vi "Set Write Mode.vi"(8 "error in (no error)":errorcluster, 10 "Write Mode":T1, 11 "Item Ref in":T2 format="%.0x") -> (0 "error out":errorcluster, 3 "Item Ref out":T2 format="%.0x")   [LabVIEW 2020, in "Modbus Master System Explorer.lvlib"]
uses:
  Modbus Master System Explorer.lvlib
  <vilib>/NI VeriStand/Custom Device API/Custom Device Item Ref.ctl
  Shared/Write Mode.ctl
  Shared/Constants.vi
  <vilib>/NI VeriStand/Custom Device API/Set Item Property (U16).vi
  Shared/Modbus Master Shared.lvlib
  <vilib>/NI VeriStand/Custom Device API/Custom Device API.lvlib
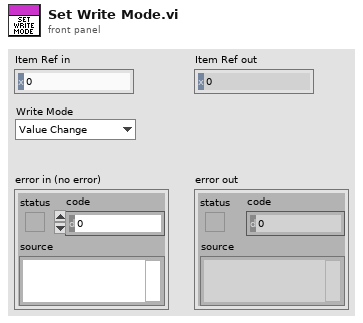
[diagram p1: front panel]
types:
  T1 = typedef "Modbus Master Shared.lvlib/Write Mode.ctl" = enum16{"Value Change", "Interval"}
  T2 = typedef "Custom Device API.lvlib/Custom Device Item Ref.ctl" = u64
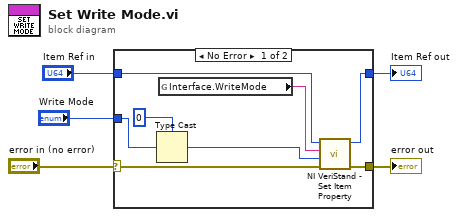
[diagram p0: block diagram]
diagram:
  n1 = case shown="No Error" "error in (no error)" {
    selector: "error in (no error)" -> [w12 w14]
    tunnel: "Item Ref in" -> [w11 w15]
    tunnel: [w10 w14] -> w3
    tunnel: [w9 w15] -> w2
    tunnel: "Write Mode" -> [w7 _]
    frame No Error {
      n2 = Type Cast(type=u16 0 ("Value"), x=w7) -> (*(type *) &x=w6:u16)
      n3 = global read "Constants.vi" "Interface.WriteMode"() -> (w13:string)
      n4 = call-poly <vilib>:"NI VeriStand - Set Item Property.vi"("error in (no error)"=w12, "Value"=w6, "Property Name"=w13, "Item Ref in"=w11) -> ("error out"=w10:errorcluster, "Item Ref out"=w9:T2)  [unwired: 5 in, 1 out]
    }
    frame Error {
    }
  }
  "error out" <- w3
  "Item Ref out" <- w2
